vi "Get Readout Modes.vi"(8 "error in (no error)":errorcluster, 11 "Camera in":refnum<class "Camera.lvclass">) -> (0 "error out":errorcluster, 3 "Camera out":refnum<class "Camera.lvclass">)   [LabVIEW 2023, in "Camera.lvlib" / "Camera.lvclass"]
uses:
  Camera.lvclass
  Camera.lvclass/Camera.ctl
  <vilib>/ActorFramework/Actor/Actor.lvclass
  Application Messages/Update Camera Modes Msg/Update Camera Modes Msg.lvclass
  C:/FlashGordon/Development/Hardware/Device/Device.lvclass
  C:/Program Files/National Instruments/LabVIEW 2023/vi.lib/ActorFramework/Actor/Actor.lvclass
  C:/FlashGordon/Development/Hardware/Camera/Camera.lvclass
panel:
  out "StringsAndValues":cluster{"String":string, "Value":i32}[](array[cluster])
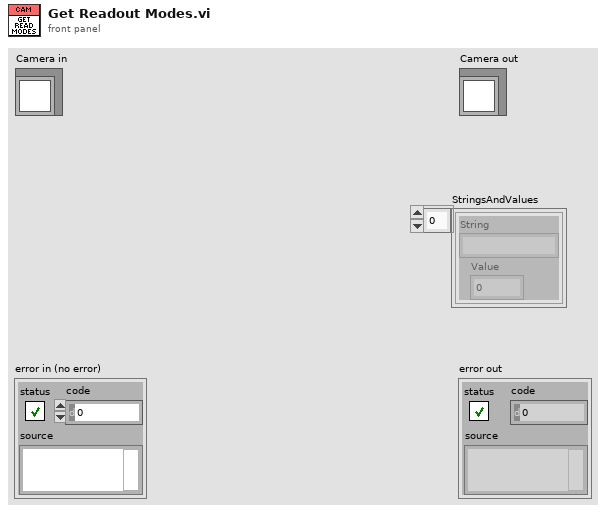
[diagram p1: front panel]
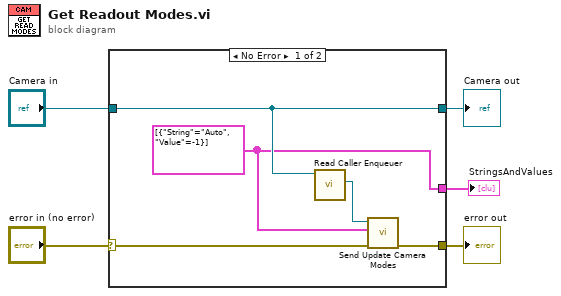
[diagram p0: block diagram]
diagram:
  n1 = case shown="No Error" "error in (no error)" {
    selector: "error in (no error)" -> [w8 w12]
    tunnel: [w7 w12] -> w4
    tunnel: [w10 w11] -> w2
    tunnel: "Camera in" -> [w10 w11]
    tunnel: [w6 _] -> w1
    frame No Error {
      w6 = cluster{"String":string, "Value":i32}[] [{"String"="Auto", "Value"=-1}] ("StringsAndValues")
      n2 = call <vilib>:"Read Caller Enqueuer.vi"("Actor"=w10) -> ("Caller Enqueuer"=w9:refnum<class "Message Enqueuer.lvclass">)  [unwired: 10 in]
      n3 = call "Send Update Camera Modes.vi"("error in (no error)"=w8, "StringsAndValues"=w6, "Message Enqueuer"=w9) -> ("error out"=w7:errorcluster)  [unwired: 7 in, 1 out]
    }
    frame Error {
    }
  }
  "error out" <- w4
  "Camera out" <- w2
  "StringsAndValues" <- w1
